vi "First-Order Hold.vi"   [LabVIEW 2020, in "NI_AdvCtrl_discrete linear.lvlib"]
doc: "LabVIEW no longer supports this VI. You can obtain similar functionality by installing the LabVIEW Simulation Module.\n\nA first-order sample and hold predicts the value of the output based on the first derivative of a given input signal."
uses:
  <vilib>/addons/control/advanced/NI_AdvCtrl_discrete linear.lvlib
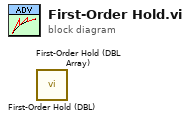
[diagram p0: block diagram]
diagram:
  n1 = call <vilib>:"First-Order Hold (DBL).vi"() -> ()  [unwired: 5 in, 1 out]
  n2 = call <vilib>:"First-Order Hold (DBL Array).vi"() -> ()  [unwired: 5 in, 1 out]
